vi "Start Search.vi"(8 "error in (no error)":errorcluster, 9 "Progress WD":refnum<user-event>, 10 "New Result Event":refnum<user-event>, 11 "Search in":refnum<class "Search.lvclass">) -> (0 "error out":errorcluster, 3 "Search out":refnum<class "Search.lvclass">)   [LabVIEW 2016, in "Better Search.lvlib" / "Search.lvclass"]
uses:
  Search.lvclass
  Search Result/Search Result.lvclass
  BetterSearch/Search Result.ctl
  Better Search.lvlib
  Search Progress.ctl
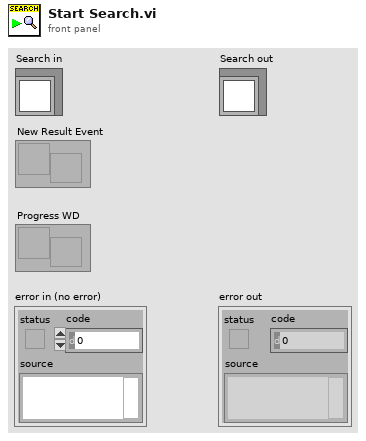
[diagram p1: front panel]
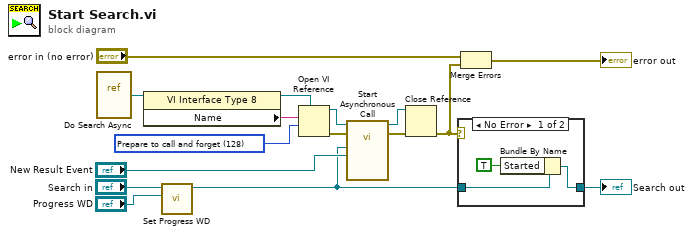
[diagram p0: block diagram]
diagram:
  w10 = 128 items=["Record modifications"=1, "Open templates for editing"=2, "Prompt user to save"=4, "Prepare for reentrant run"=8, "Prompt to find missing subVIs"=16, "Hide loading dialog box"=32, "Enable simultaneous calls"=64, "Prepare to call and forget"=128, "Simultaneous call and forget"=192, "Prepare to call and collect"=256, "Simultaneous call and collect"=320]
  n1 = vi-ref "Do Search Async.vi"() -> (w8:refnum<vi>)
  n2 = property class="VI Interface Type 8"(reference=w8) -> (reference out=w11:refnum<vi>, "Name"=w9:string)  [unwired: 1 in, 1 out]
  n3 = call "Set Progress WD.vi"("Progress WD"="Progress WD", "Search in"="Search in") -> ("Search out"=w2:refnum<class "Search.lvclass">)  [unwired: 8 in, 1 out]
  n4 = Open VI Reference(type specifier VI Refnum (for type only)=w11, vi path=w9, options=w10) -> (vi reference=w13:refnum<vi>, error out=w12:errorcluster)  [unwired: 3 in]
  n5 = call-by-ref "Start Asynchronous Call"(reference=w13, error in=w12, "New Result Event"="New Result Event", "Search in"=w2) -> (reference out=w15:refnum<vi>, error out=w14:errorcluster)  [unwired: 10 in]
  n6 = Close Reference(reference=w15, error in (no error)=w14) -> (error out=w5:errorcluster)
  n7 = case shown="No Error" w5 {
    tunnel: w2 -> [w19 w20]
    tunnel: [w17 w20] -> w4
    frame No Error {
      n8 = Bundle By Name(cluster=w19, "Started"=TRUE) -> (w17:refnum<class "Search.lvclass">)
    }
    frame Error {
    }
  }
  "Search out" <- w4
  n9 = Merge Errors("error in (no error)", w5) -> (→"error out":errorcluster)
